vi "SettingManagerRunVI.vi"(8 "error in (no error)":errorcluster, 11 "VI in":refnum<vi>) -> (0 "error out":errorcluster, 3 "VI out":refnum<vi>)   [LabVIEW 2021]
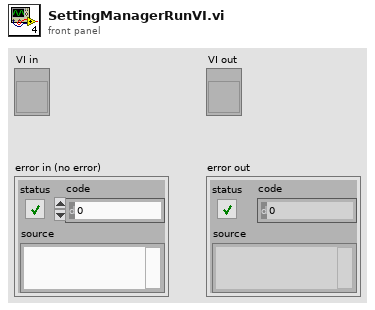
[diagram p1: front panel]
types:
  T1 = enum32{"Bad", "Idle", "Run top level", "Running"}
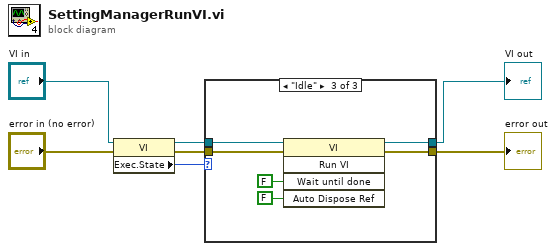
[diagram p0: block diagram]
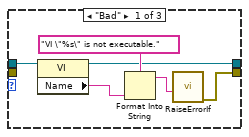
[diagram p2: hidden frame]
diagram:
  n1 = property class="VI"(reference="VI in", error in="error in (no error)") -> (reference out=w5:refnum<vi>, error out=w3:errorcluster, "Exec.State"=w6:T1)
  n2 = case shown="\"Idle\"" w6 {
    tunnel: w5 -> [w13 w15 w21]
    tunnel: w3 -> [_ w14 w20]
    tunnel: [w8 w15 w17] -> w2
    tunnel: [w9 w14 w16] -> w1
    frame "Bad" {
      n3 = property class="VI"(reference=w13) -> (reference out=w8:refnum<vi>, "Name"=w11:string)  [unwired: 1 in, 1 out]
      n4 = Format Into String(format string="VI \"%s\" is not executable.", w11) -> (resulting string=w10:string)  [unwired: 2 in, 1 out]
      n5 = call "RaiseErrorIf.vi"("error message"=w10) -> ("error out"=w9:errorcluster)  [unwired: 10 in]
    }
    frame Default {
    }
    frame "Idle" {
      n6 = invoke class="VI" method="Run VI"(reference=w21, error in=w20, "Wait until done"=FALSE ("Wait Until Done"), "Auto Dispose Ref"=FALSE ("Auto Dispose Reference")) -> (reference out=w17:refnum<vi>, error out=w16:errorcluster)  [unwired: 1 in, 3 out]
    }
  }
  "VI out" <- w2
  "error out" <- w1
